vi "Game_InitializeMap.vi"(2 "NrOfPlayers":T1) -> ()   [LabVIEW 2018]
uses:
  TypDefs/Player_Enum.ctl
  <vilib>/rvi/DataTransferAndStorage/Container/Common/niFpgaContainerExecOnDevCompGetState.vi
  <vilib>/rvi/Emulation/niFpgaEmulationIsFPGAContextNoSignature.vi
  <vilib>/rvi/DataTransferAndStorage/Container/Common/niFpgaContainerGetUniqueNameForEmu.vi
  <vilib>/rvi/Emulation/niFpgaProcessEmulError.vi
  <vilib>/rvi/Emulation/niFpgaSctlEmulationGetInTimedLoop.vi
  <vilib>/rvi/errors/nirviReportUnexpectedCaseInternalError (U32).vi
  <vilib>/rvi/Memory/Memory_Emulation/niFpgaMemoryEmulationCacheClearOnFirstRun.vi
  <vilib>/rvi/Memory/Memory_Emulation/nirvimemoryEmulationManagerCache_MakeExclusive.vi
  <vilib>/rvi/Memory/Memory_Emulation/niFpgaMemoryEmulationValidateCache.vi
  <vilib>/rvi/Memory/Memory_Emulation/nirvimemoryEmulationManagerCache_InsertValue.vi
  <vilib>/Utility/error.llb/Clear Errors.vi
  <vilib>/rvi/Memory/Memory_Emulation/nirvimemoryEmulationManagerCache_ReleaseExclusive.vi
  <vilib>/rvi/Memory/Memory_Emulation/nirvimemoryEmulationManagerCache_GetValue.vi
  <vilib>/rvi/Memory/Memory_Emulation/nirvimemoryEmulationManagerCache_SetValue.vi
  <vilib>/rvi/Emulation/niFpgaSctlEmulationResourceMgr.vi
  <vilib>/rvi/DataTransferAndStorage/Container/XNode/niFpgaContainer.xnode
  <vilib>/rvi/Memory/Memory_Emulation/niFpgaMemoryEmulationRefIn.vi
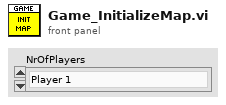
[diagram p1: front panel]
types:
  T1 = typedef "Player_Enum.ctl" = enum16{"Player 1", "Player 2"}
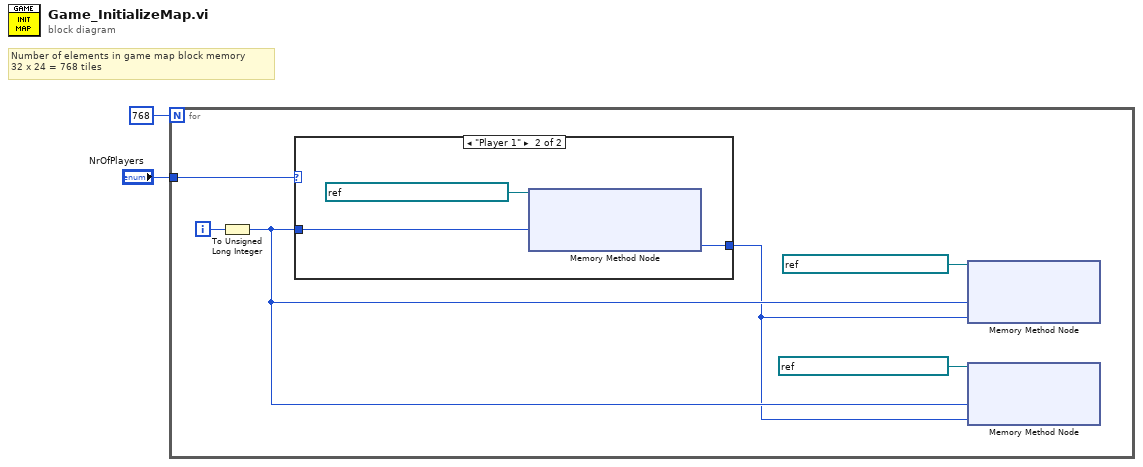
[diagram p0: block diagram]
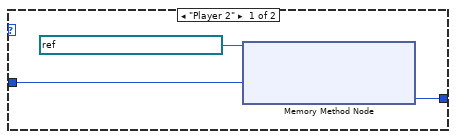
[diagram p2: hidden frame]
diagram:
  # "Number of elements in game map block memory\n32 x 24 = 768 tiles"
  n1 = for {
    N: 768 -> [_]
    tunnel: "NrOfPlayers" -> [w3]
    i -> [w8]
    n2 = To Unsigned Long Integer(number=w8) -> (unsigned 32bit integer=w7:u32)
    n3 = case shown="\"Player 1\"" w3 {
      tunnel: w7 -> [w11 w14]
      tunnel: [w10 w13] -> w6
      frame "Player 2" {
        n4 = xnode ("Memory Method Node")("Address"=w11, "Memory In"=refnum<k21> "BlockMem_2PlayerGameMap") -> ("Data"=w10:u8)  [unwired: 1 out]
      }
      frame "Player 1" {
        n5 = xnode ("Memory Method Node")("Address"=w14, "Memory In"=refnum<k21> "BlockMem_1PlayerGameMap") -> ("Data"=w13:u8)  [unwired: 1 out]
      }
    }
    n6 = xnode ("Memory Method Node")("Address"=w7, "Data"=w6, "Memory In"=refnum<k21> "BlockMem_FastGameMap") -> ()  [unwired: 1 out]
    n7 = xnode ("Memory Method Node")("Address"=w7, "Data"=w6, "Memory In"=refnum<k21> "BlockMem_SlowGameMap") -> ()  [unwired: 1 out]
  }
